vi "LS218_INIT_TABLEAU_MESURES.vi"(8 "error in (no error)":errorcluster caption="entrée d'erreur (pas d'erreur)", 10 "Voies de mesures":T2(array[cluster])) -> (0 "error out":errorcluster caption="sortie d'erreur", 2 "table_acq":T1(array[cluster]))   [LabVIEW 2016]
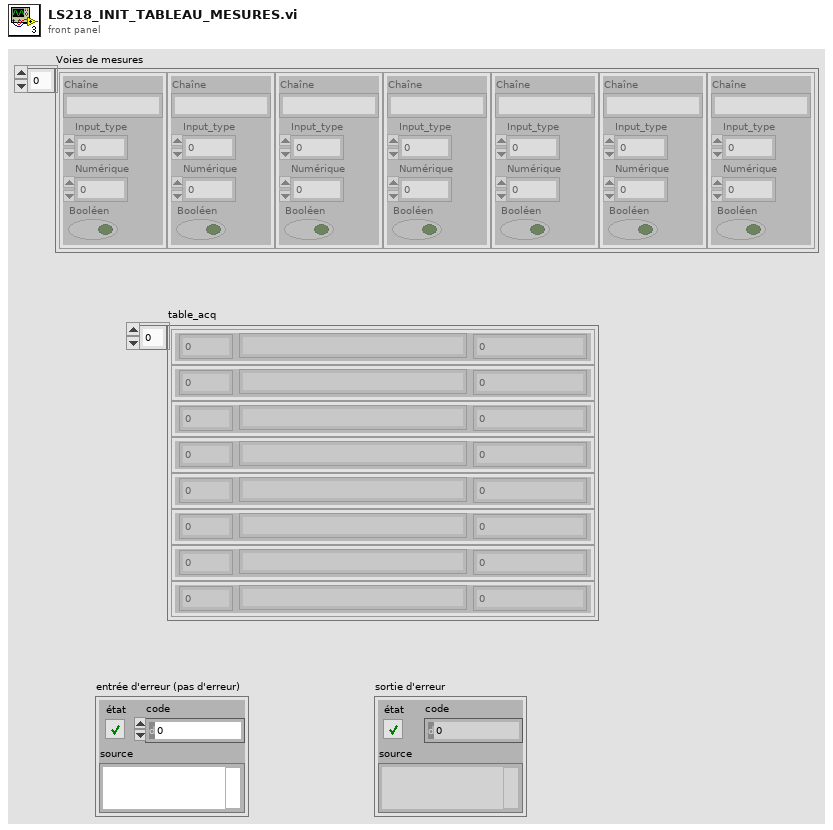
[diagram p1: front panel]
types:
  T1 = cluster{"N_voie":i32, "Nom_voie":string, "Mesure_voie":dbl}[]
  T2 = cluster{"Chaîne":string, "Input_type":u16, "Numérique":dbl, "Booléen":bool}[]
  T3 = cluster{"N_voie":i32, "Nom_voie":string, "Mesure_voie":dbl}
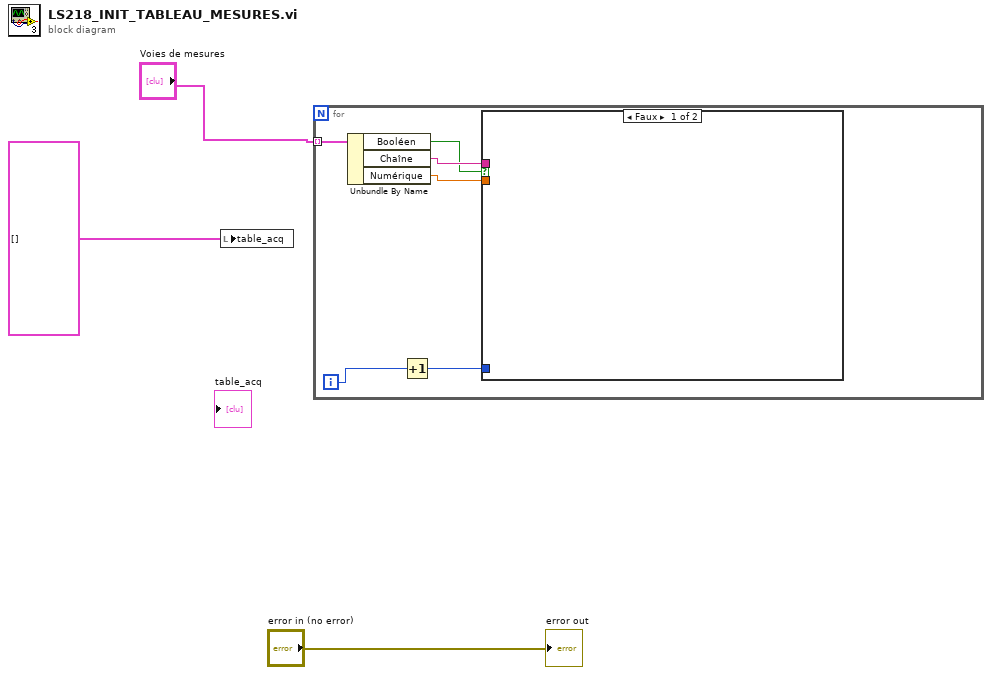
[diagram p0: block diagram]
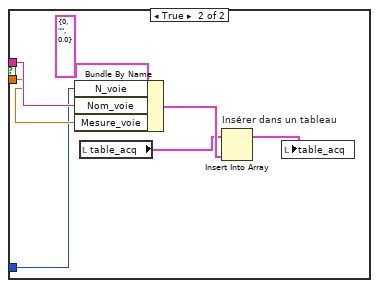
[diagram p2: hidden frame]
diagram:
  n1 = local write "table_acq"(T1 [] ("table_acq")) -> ()
  n2 = for {
    tunnel: "Voies de mesures" -> [w9] mode=indexing
    i -> [w5]
    n3 = Unbundle By Name(w9) -> ("Booléen"=w6:bool, "Chaîne"=w8:string, "Numérique"=w7:dbl)
    n4 = Increment(x=w5) -> (x+1=w4:i32)
    n5 = case shown="Faux" w6 {
      tunnel: w8 -> [_ w15]
      tunnel: w7 -> [_ w14]
      tunnel: w4 -> [_ w13]
      frame False {
      }
      frame True {
        n6 = Bundle By Name(cluster=T3 {"N_voie"=0, "Nom_voie"="", "Mesure_voie"=0.0} ("Tableau_acq"), "N_voie"=w13, "Nom_voie"=w15, "Mesure_voie"=w14) -> (w12:T3)
        n7 = local read "table_acq"() -> (w10:T1)
        n8 = Insert Into Array "Insérer dans un tableau"(array=w10, new element=w12) -> (w11:T1)  [unwired: 1 in]
        n9 = local write "table_acq"(w11) -> ()
      }
    }
  }
  "error out" <- "error in (no error)"
